vi "Configure Frequency Domain Averaging.vi"(6 "Frequency Trigger Delay (0 s)":dbl, 7 "Frequency Number Of Averages (1)":i32=1, 8 "error in (no error)":errorcluster, 9 "Frequency Averaging (0: avgNone)":i32(ring) items=["avgNone", "avgFixedLength", "avgContinuous", "avgPeakFixedLength", "avgPeakContinuous"], 10 "Analyzer (0: A0)":i32(ring) items=["A0", "A1"], 11 "VISA resource name":refnum<visa-resource-name>) -> (0 "error out":errorcluster, 3 "VISA resource name out":refnum<visa-resource-name>)   [LabVIEW 2014, in "Stanford Research SR1.lvlib"]
doc: "Configures the attributes for the Frequency Domain Averaging."
uses:
  Stanford Research SR1.lvlib
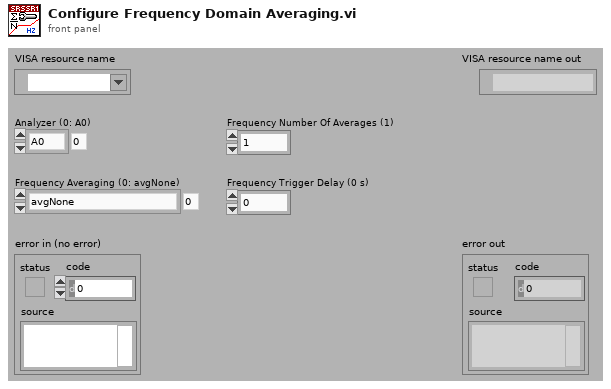
[diagram p1: front panel]
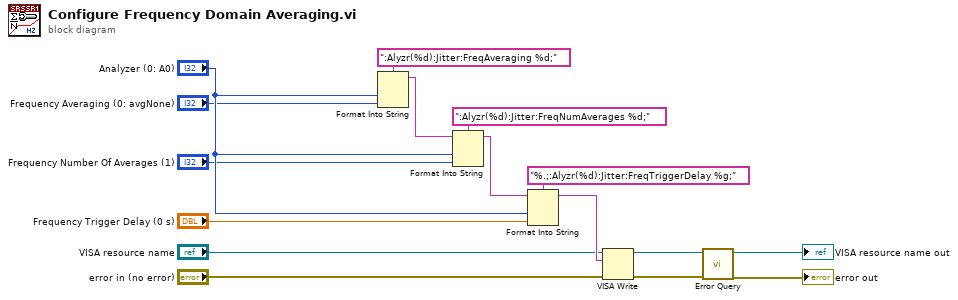
[diagram p0: block diagram]
diagram:
  n1 = Format Into String(format string=":Alyzr(%d):Jitter:FreqAveraging %d;", "Analyzer (0: A0)", "Frequency Averaging (0: avgNone)") -> (resulting string=w15:string)  [unwired: 2 in, 1 out]
  n2 = Format Into String(format string=":Alyzr(%d):Jitter:FreqNumAverages %d;", initial string=w15, "Analyzer (0: A0)", "Frequency Number Of Averages (1)") -> (resulting string=w13:string)  [unwired: 1 in, 1 out]
  n3 = Format Into String(format string="%.;:Alyzr(%d):Jitter:FreqTriggerDelay %g;", initial string=w13, "Analyzer (0: A0)", "Frequency Trigger Delay (0 s)") -> (resulting string=w11:string)  [unwired: 1 in, 1 out]
  n4 = VISA Write(VISA resource name="VISA resource name", write buffer=w11, error in (no error)="error in (no error)") -> (VISA resource name out=w8:refnum<visa-resource-name>, error out=w7:errorcluster)  [unwired: 1 out]
  n5 = call "Error Query.vi"("error in (no error)"=w7, "VISA resource name"=w8) -> ("error out"=→"error out":errorcluster, "VISA resource name out"=→"VISA resource name out":refnum<visa-resource-name>)  [unwired: 6 in, 2 out]
